vi "GT Set Laser Crd Map.vi"(8 "error in (no error)":errorcluster caption="错误输入（无错误）", 9 "map":i16, 10 "channel":i16, 11 "cardNum":i16) -> (0 "error out":errorcluster caption="错误输出", 3 "function return":i16)   [LabVIEW 2020, in "gts.lvlib"]
doc: "GT_API GT_SetLaserCrdMap(short cardNum,short channel,short map);"
uses:
  gts.lvlib
  dll/32bit/multi_card/gts.dll
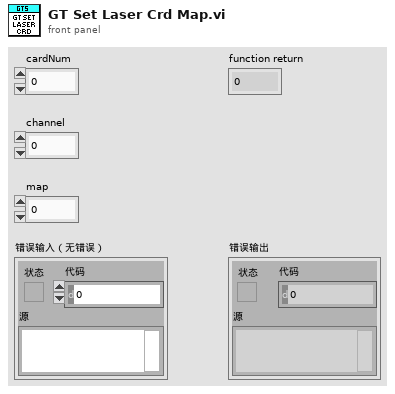
[diagram p1: front panel]
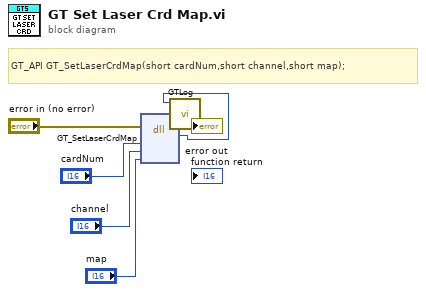
[diagram p0: block diagram]
diagram:
  # "GT_API GT_SetLaserCrdMap(short cardNum,short channel,short map);"
  n1 = dll-call lib="C:/1228/dll/32bit/multi_card/gts.dll" fn="GT_SetLaserCrdMap"(error in="error in (no error)", "cardNum"="cardNum", "channel"="channel", "map"="map") -> (error out=w3:errorcluster, w1:i16)  [unwired: 5 in, 1 out]
  n2 = call "GTLog.vi"("error in (no error)"=w3, "Numeric"=w1) -> ("error out"=→"error out":errorcluster)  [unwired: 9 in]
